vi "Run1TonNew.vi"() -> ()   [LabVIEW 2014]
doc: "Use this template to build a producer/consumer design pattern with events to produce queue items. Use this design pattern instead of the User Interface Event Handler pattern for user interfaces when you want to execute code asynchronously in response to an event without slowing the user interface responsiveness."
uses:
  <vilib>/addons/h5labview2/base/hid_t.ctl
  DatasetNames.ctl
  Program Files (x86)/CAEN/Comm/labview/CAENComm.lvlib
panel:
  out "Time Data (E-4 s)":T1
  in  "Monitoring Delay (ms)":u16=100 caption="Monitoring Delay (ms) (TDC, QDC, Dig, Time)"
  out "Duty Factor":dbl(graph)
  in  "?":T2(tab)
  out "TDC Histograms":u16[][](graph)
  out "QDC Histograms":u16[][](graph)
  out "Digitizer 1":dbl[][](graph)
  out "Scaler Rates":T3(graph)
  in  "Scaler Delay (s)":sgl=10.0
  out "Time Histogram":u16[][](graph)
  in  "Max Hist Time (s)":sgl=0.25 format="%#_13g"
  in  "Time # Bins":i32=1000
  out "Temp Chart":dynamicdata(graph)
  out "Total Samples":sgl caption="Number of Samples Being Averaged"
  out "Mean":sgl
  in  "Temp Delay (s)":sgl=1.0
  in  "Max Samples":u32=600
  out "# elements in queue":i32
  out "Acquiring?":bool
  out "Scaler Data":u32[](array[numeric])
  out "Acquisition\nErrors":errorcluster
  in  "Clear Acquisition Errors":bool
  in  "QDC threshold":u16=1
  in  "Start Acquisition":bool
  out "# Events Written":i32
  in  "# Events to\nRecord":i32
  out "Analysis\nErrors":errorcluster
  in  "Calibrate Verniers":bool
  in  "Stop Acquisition":bool
  in  "Configure Output":bool
  in  "Calibrate Pedestals":bool
  in  "stop":bool
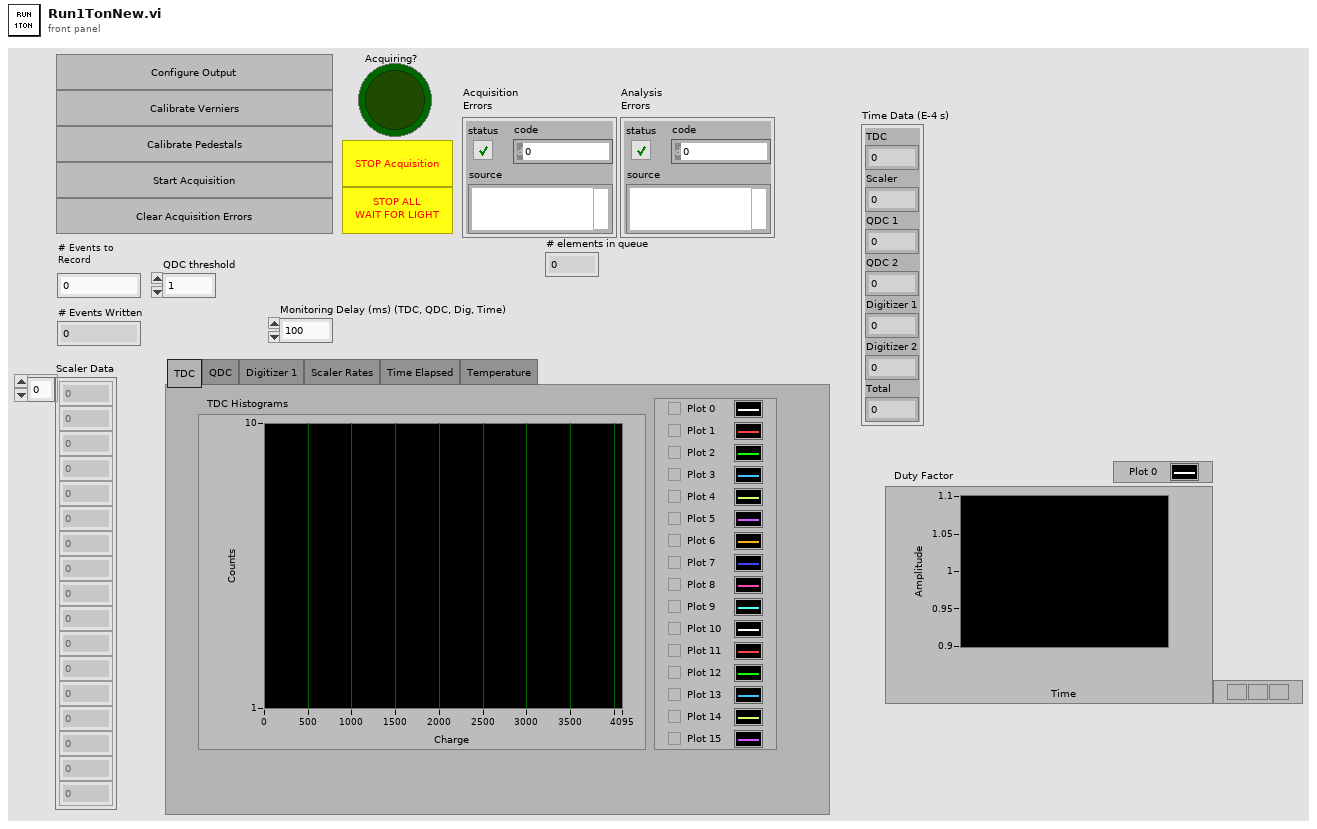
[diagram p1: front panel]
types:
  T1 = cluster{"TDC":u16, "Scaler":u16, "QDC 1":u16, "QDC 2":u16, "Digitizer 1":u16, "Digitizer 2":u16, "Total":u16}
  T2 = enum32{"TDC", "QDC", "Digitizer 1", "Scaler Rates", "Time Elapsed", "Temperature"}
  T3 = cluster{"[0]":dbl, "[1]":dbl, "[2]":dbl, "[3]":dbl}
  T4 = typedef "hid_t.ctl" = i32
  T5 = cluster{"State":enum16{"Startup", "Initialise", "Event OK", "Discard Event", "Exit", "Close"}, "Data":variant}
  T6 = typedef "DatasetNames.ctl" = enum16{"TDC", "Scaler", "QDC_1", "QDC_2", "Digitizer_1", "Digitizer_2", "Event_Time", "Event_Temp"}
  T7 = cluster{"TDC Data":u32[], "Scaler Data":u32[], "QDC 1 Data":u32[], "QDC 2 Data":u32[], "Digitizer 1 TRIG_REC":u32, "Digitizer 1 Waveforms":u32[], "Digitizer 2 TRIG_REC":u32, "Digitizer 2 Waveforms":u32[], "Event Start UNIX Time":dbl}
  T8 = enum16{"Startup", "Initialise", "Event OK", "Discard Event", "Exit", "Close"}
  T9 = cluster{"[0]":dbl, "[1]":dbl, "[2]":dbl, "[3]":dbl}[]
  T10 = cluster{"Channel":u8, "QDC Data":u16, "LowRange?":bool}[]
  T11 = cluster{"Data out[0]":u16, "Data out[1]":u16, "Data out[2]":u16, "Data out[3]":u16, "Data out[4]":u16, "Data out[5]":u16, "Data out[6]":u16}
  T12 = enum16{"Configure", "Initialise", "Run", "Close"}
  T13 = cluster{"TDC":u32, "Scaler":u32, "QDC 1":u32, "QDC 2":u32, "Digitizer 1":u32, "Digitizer 2":u32}
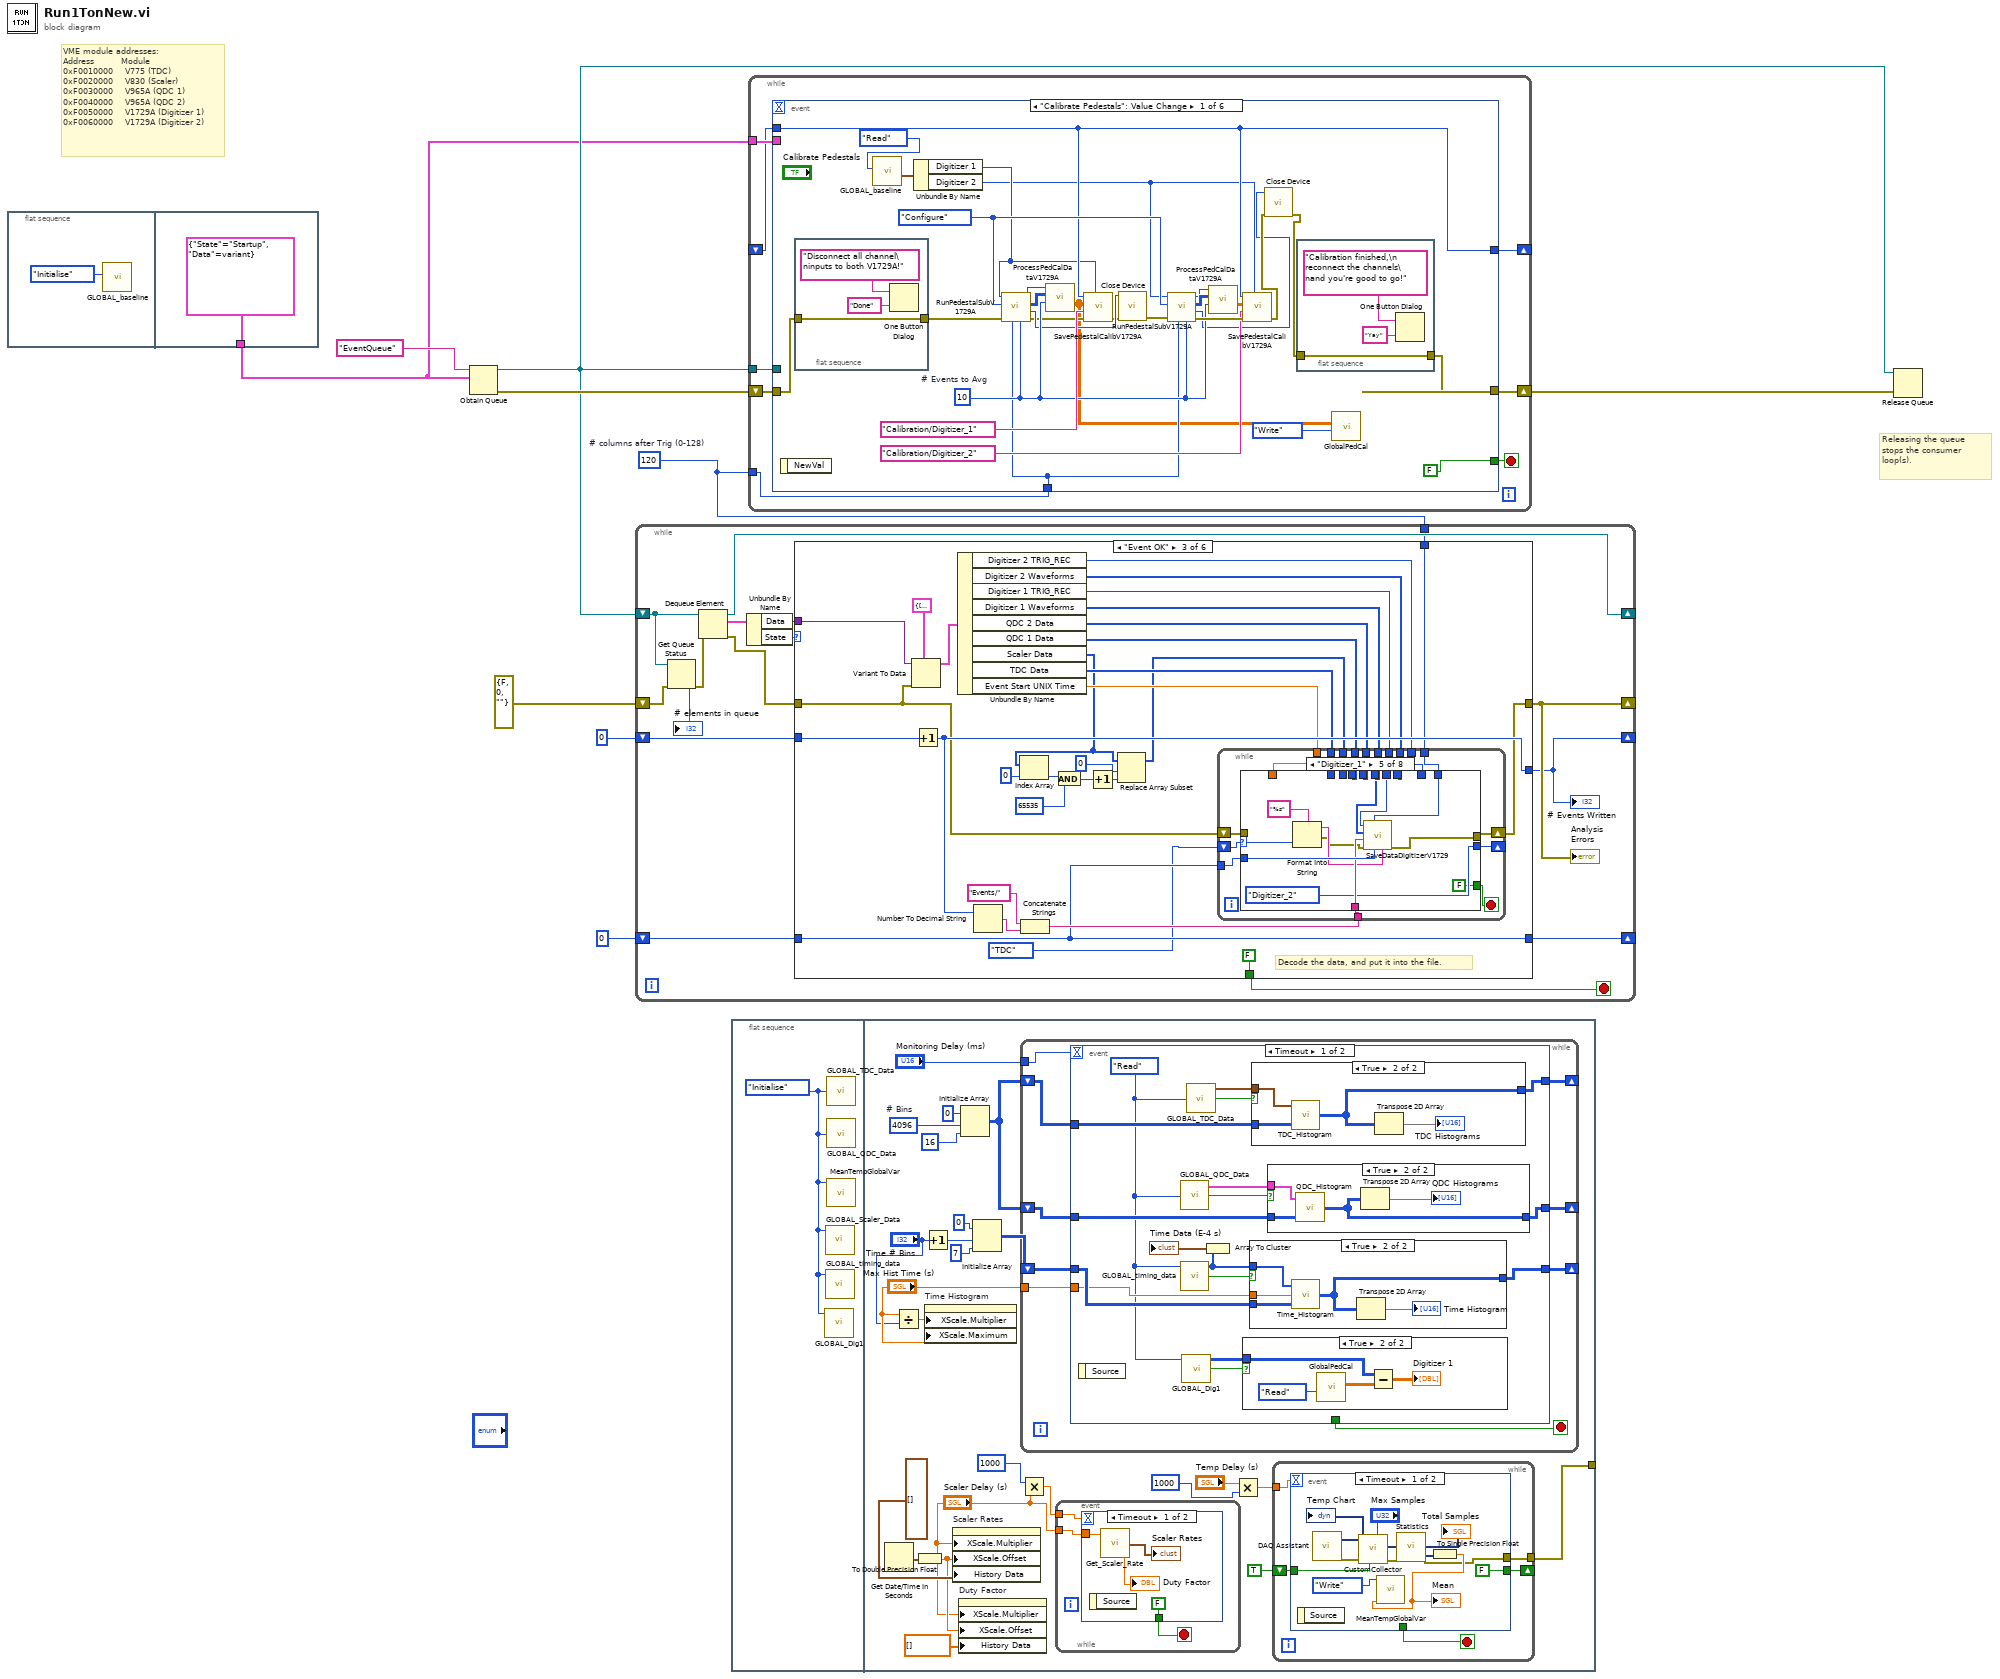
[diagram p0: block diagram]
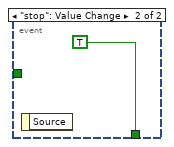
[diagram p2: hidden frame]
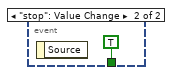
[diagram p3: hidden frame]
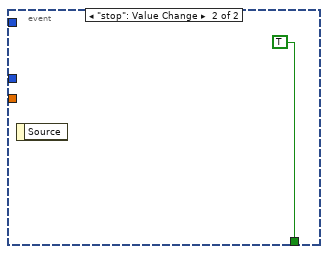
[diagram p8: hidden frame]
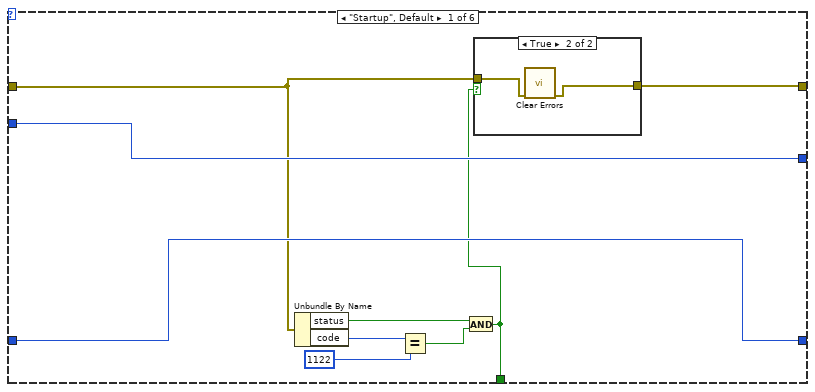
[diagram p9: hidden frame]
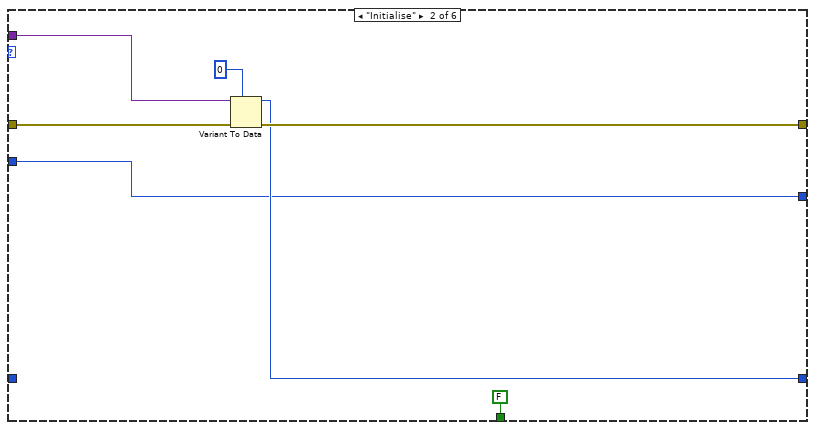
[diagram p11: hidden frame]
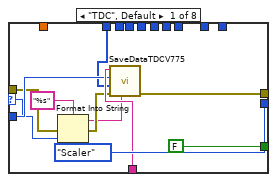
[diagram p12: hidden frame]
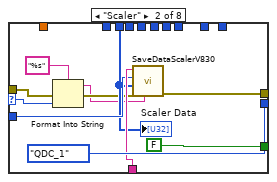
[diagram p13: hidden frame]
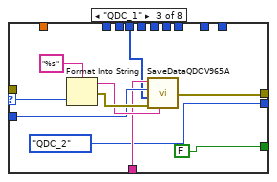
[diagram p14: hidden frame]
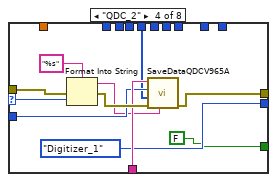
[diagram p15: hidden frame]
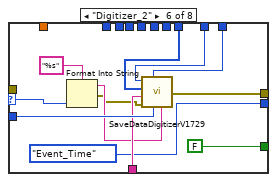
[diagram p16: hidden frame]
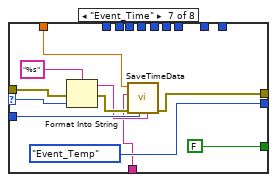
[diagram p17: hidden frame]
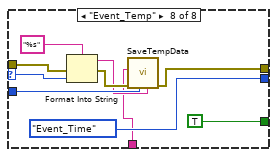
[diagram p18: hidden frame]
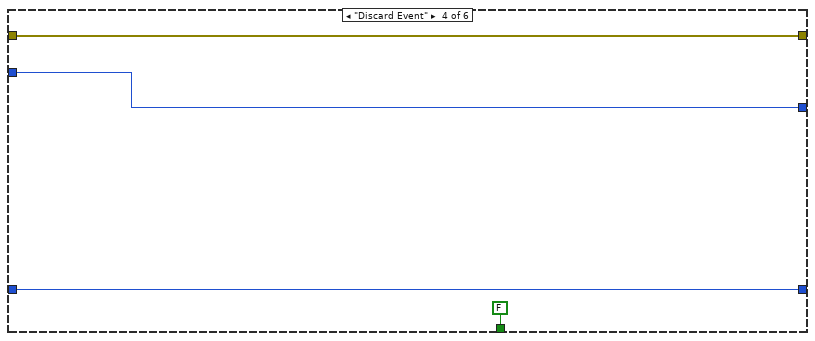
[diagram p19: hidden frame]
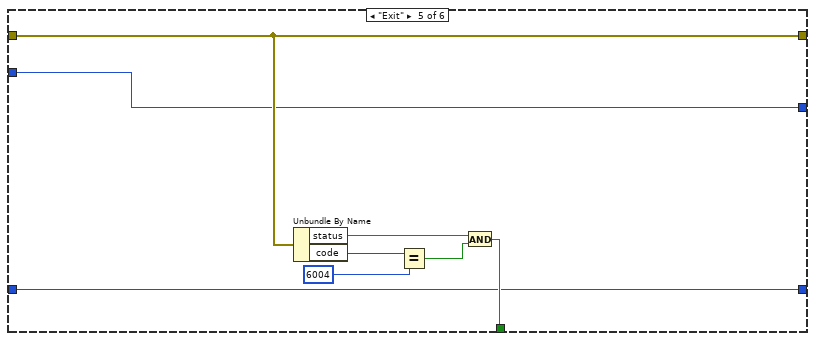
[diagram p20: hidden frame]
diagram:
  w1 = u16 120  # # columns after Trig (0-128)
  # "VME module addresses:\nAddress         Module\n0xF0010000    V775 (TDC)\n0xF0020000    V830 (Scaler)\n0xF0030000    V965A (QDC 1)\n0xF0040000    V965A (QDC 2)\n0xF0050000    V1729A (Digitizer 1)\n0xF0060000    V1729A (Digitizer 2)"
  # "Releasing the queue stops the consumer loop(s)."
  n1 = flat-sequence {
    tunnel: [T5 {"State"=enum."Startup", "Data"=variant}] -> w2
    frame #0 {
      n2 = call "GLOBAL_baseline.vi"("State"=enum16{"Initialise", "Write", "Read"}."Initialise") -> ()  [unwired: 10 in, 1 out]
    }
    frame #1 {
    }
  }
  n3 = Obtain Queue(name (unnamed)="EventQueue", element data type=w2) -> (queue out=w4:refnum<queue>, error out=w9:errorcluster)  [unwired: 3 in, 1 out]
  n4 = while {
    shift-right: [w17] -> _
    shift-left: errorcluster {"status"=FALSE, "code"=0, "source"=""} ("error out") -> [w15]
    shift-right: [w23] -> _
    shift-left: w4 -> [w13]
    shift-right: [w21] -> _
    shift-left: T4 0 ("File Handle") -> [w20]
    tunnel: w1 -> [w19]
    shift-right: [w16] -> _
    shift-left: 0 -> [w18]
    stop <- w22 stop-if-true
    n5 = Get Queue Status(queue=w13, error in (no error)=w15) -> (error out=w14:errorcluster, # elements in queue=→"# elements in queue":i32)  [unwired: 1 in, 6 out]
    n6 = Dequeue Element(queue=w13, error in (no error)=w14) -> (queue out=w23:refnum<queue>, element=w27:T5, error out=w24:errorcluster)  [unwired: 1 in, 1 out]
    n7 = Unbundle By Name(w27) -> ("Data"=w25:variant, "State"=w26:T8)
    n8 = case shown="\"Event OK\"" w26 {
      tunnel: w25 -> [_ w44 w75 _ _ _]
      tunnel: w24 -> [w30 w43 w62 w185 w188 w197]
      tunnel: [w28 w42 w60 w185 w188 w197] -> w17
      tunnel: [w29 FALSE FALSE FALSE w189 FALSE] -> w22
      tunnel: [w32 w41 w65 w183 w187 w195] -> w21
      tunnel: w20 -> [w32 _ w65 w183 w187 w195]
      tunnel: w19 -> [_ _ w67 _ _ _]
      tunnel: w18 -> [w31 w40 w74 w182 w186 w194]
      tunnel: [w31 w40 w73 w182 w186 w194] -> w16
      frame "Startup", Default {
        n9 = Unbundle By Name(w30) -> ("status"=w36:bool, "code"=w34:i32)
        n10 = Equal?(x=w34, y=1122) -> (x = y?=w35:bool)
        n11 = And(x=w36, y=w35) -> (x .and. y?=w29:bool)
        n12 = case shown="True" w29 {
          tunnel: w30 -> [w37 w39]
          tunnel: [w37 w38] -> w28
          frame False {
          }
          frame True {
            n13 = call <vilib>:"Clear Errors.vi"("error in (no error)"=w39) -> ("error out"=w38:errorcluster)  [unwired: 5 in, 1 out]
          }
        }
      }
      frame "Initialise" {
        n14 = Variant To Data(error in=w43, type=T4 0 ("File Handle"), Variant=w44) -> (data=w41:T4, error out=w42:errorcluster)
      }
      frame "Event OK" {
        # "Decode the data, and put it into the file."
        n15 = Variant To Data(error in=w62, type=T7 {"TDC Data"=[], "Scaler Data"=[], "QDC 1 Data"=[], "QDC 2 Data"=[], "Digitizer 1 TRIG_REC"=0, "Digitizer 1 Waveforms"=[], "Digitizer 2 TRIG_REC"=0, "Digitizer 2 Waveforms"=[], "Event Start UNIX Time"=0.0}, Variant=w75) -> (data=w69:T7)  [unwired: 1 out]
        n16 = Increment(x=w74) -> (x+1=w73:i32)
        n17 = Unbundle By Name(w69) -> ("Digitizer 2 TRIG_REC"=w68:u32, "Digitizer 2 Waveforms"=w55:u32[], "Digitizer 1 TRIG_REC"=w57:u32, "Digitizer 1 Waveforms"=w58:u32[], "QDC 2 Data"=w64:u32[], "QDC 1 Data"=w63:u32[], "Scaler Data"=w51:u32[], "TDC Data"=w61:u32[], "Event Start UNIX Time"=w56:dbl)
        n18 = Number To Decimal String(number=w73) -> (decimal integer string=w71:string)  [unwired: 1 in]
        n19 = Index Array(array=w51, index=0) -> (element=w53:u32)
        n20 = Concatenate Strings("Events/", w71) -> (w66:string)
        n21 = And(x=w53, y=u32 65535) -> (x .and. y?=w50:u32)
        n22 = Increment(x=w50) -> (x+1=w47:u32)
        n23 = Replace Array Subset(array=w51, new element=w47, index=0) -> (w48:u32[])
        n24 = while {
          tunnel: w68 -> [w93]
          tunnel: w55 -> [w92]
          tunnel: w67 -> [w91]
          tunnel: w66 -> [w90]
          tunnel: w65 -> [w89]
          tunnel: w57 -> [w88]
          tunnel: w58 -> [w87]
          tunnel: w64 -> [w85]
          tunnel: w63 -> [w84]
          shift-right: [w81] -> w60
          shift-left: w62 -> [w86]
          tunnel: w48 -> [w83]
          tunnel: w61 -> [w82]
          shift-right: [w80] -> _
          shift-left: DatasetNames."TDC" -> [w79]
          tunnel: w56 -> [w77]
          stop <- w78 stop-if-true
          n25 = case shown="\"Digitizer_1\"" w79 {
            selector: w79 -> [w94 w108 w122 w135 w144 w153 w170 w180]
            tunnel: [w102 w113 w119 w128 w148 w160 w164 w174] -> w81
            tunnel: w93 -> [_ _ _ _ _ w159 _ _]
            tunnel: w92 -> [_ _ _ _ _ w158 _ _]
            tunnel: w89 -> [w100 w111 w121 w131 w147 w157 w165 w175]
            tunnel: w91 -> [_ _ _ _ w146 w156 _ _]
            tunnel: w90 -> [w101 w112 w120 w132 w145 w155 w162 w172]
            tunnel: w88 -> [_ _ _ _ w140 _ _ _]
            tunnel: w87 -> [_ _ _ _ w139 _ _ _]
            tunnel: w86 -> [w97 w107 _ w134 _ _ w167 w177]
            tunnel: w85 -> [_ _ _ w130 _ _ _ _]
            tunnel: w84 -> [_ _ w118 _ _ _ _ _]
            tunnel: [DatasetNames."Scaler" DatasetNames."QDC_1" DatasetNames."QDC_2" DatasetNames."Digitizer_1" DatasetNames."Digitizer_2" DatasetNames."Event_Time" DatasetNames."Event_Temp" DatasetNames."Event_Time"] -> w80
            tunnel: [FALSE FALSE FALSE FALSE FALSE FALSE FALSE TRUE] -> w78
            tunnel: w83 -> [_ w110 _ _ _ _ _ _]
            tunnel: w82 -> [w99 _ _ _ _ _ _ _]
            tunnel: w77 -> [_ _ _ _ _ _ w161 _]
            frame "TDC", Default {
              n26 = Format Into String(format string="%s", error in=w97, w94) -> (resulting string=w95:string, error out=w96:errorcluster)  [unwired: 1 in]
              n27 = call "SaveDataTDCV775.vi"("Module"=w95, "error in (no error)"=w96, "Buff"=w99, "File Handle"=w100, "String"=w101) -> ("error out"=w102:errorcluster)  [unwired: 5 in, 1 out]
            }
            frame "Scaler" {
              n28 = Format Into String(format string="%s", error in=w107, w108) -> (resulting string=w105:string, error out=w106:errorcluster)  [unwired: 1 in]
              n29 = call "SaveDataScalerV830.vi"("Module"=w105, "error in (no error)"=w106, "Buff"=w110, "File Handle"=w111, "Group Name"=w112) -> ("error out"=w113:errorcluster)  [unwired: 6 in]
              "Scaler Data" <- w110
            }
            frame "QDC_1" {
              n30 = Format Into String(format string="%s", w122) -> (resulting string=w123:string, error out=w124:errorcluster)  [unwired: 2 in]
              n31 = call "SaveDataQDCV965A.vi"("Module"=w123, "error in (no error)"=w124, "Buff"=w118, "File Handle"=w121, "String"=w120) -> ("error out"=w119:errorcluster)  [unwired: 5 in, 1 out]
            }
            frame "QDC_2" {
              n32 = Format Into String(format string="%s", error in=w134, w135) -> (resulting string=w129:string, error out=w133:errorcluster)  [unwired: 1 in]
              n33 = call "SaveDataQDCV965A.vi"("Module"=w129, "error in (no error)"=w133, "Buff"=w130, "File Handle"=w131, "String"=w132) -> ("error out"=w128:errorcluster)  [unwired: 5 in, 1 out]
            }
            frame "Digitizer_1" {
              n34 = Format Into String(format string="%s", w144) -> (resulting string=w142:string, error out=w141:errorcluster)  [unwired: 2 in]
              n35 = call "SaveDataDigitizerV1729.vi"("Module"=w142, "File Handle"=w147, "# Samples after Trig"=w146, "error in (no error)"=w141, "String"=w145, "Digitizer Waveforms"=w139, "Digitizer TRIG_REC"=w140) -> ("error out"=w148:errorcluster)  [unwired: 2 in, 2 out]
            }
            frame "Digitizer_2" {
              n36 = Format Into String(format string="%s", w153) -> (resulting string=w152:string, error out=w151:errorcluster)  [unwired: 2 in]
              n37 = call "SaveDataDigitizerV1729.vi"("Module"=w152, "File Handle"=w157, "# Samples after Trig"=w156, "error in (no error)"=w151, "String"=w155, "Digitizer Waveforms"=w158, "Digitizer TRIG_REC"=w159) -> ("error out"=w160:errorcluster)  [unwired: 2 in, 2 out]
            }
            frame "Event_Time" {
              n38 = Format Into String(format string="%s", error in=w167, w170) -> (resulting string=w163:string, error out=w166:errorcluster)  [unwired: 1 in]
              n39 = call "SaveTimeData.vi"("Module"=w163, "File Handle"=w165, "error in (no error)"=w166, "String"=w162, "Event Start UNIX Time"=w161) -> ("error out"=w164:errorcluster)  [unwired: 5 in, 1 out]
            }
            frame "Event_Temp" {
              n40 = Format Into String(format string="%s", error in=w177, w180) -> (resulting string=w173:string, error out=w176:errorcluster)  [unwired: 1 in]
              n41 = call "SaveTempData.vi"("Module"=w173, "File Handle"=w175, "error in (no error)"=w176, "String"=w172) -> ("error out"=w174:errorcluster)  [unwired: 6 in, 1 out]
            }
          }
        }
      }
      frame "Discard Event" {
      }
      frame "Exit" {
        n42 = Unbundle By Name(w188) -> ("status"=w193:bool, "code"=w191:i32)
        n43 = Equal?(x=w191, y=6004) -> (x = y?=w192:bool)
        n44 = And(x=w193, y=w192) -> (x .and. y?=w189:bool)
      }
      frame "Close" {
      }
    }
    "Analysis\nErrors" <- w17
    "# Events Written" <- w16
  }
  n45 = flat-sequence {
    tunnel: [w199] -> _
    frame #0 {
      w198 = enum16{"Initialise", "Write", "Read"}."Initialise" ("State")
      n46 = call "GLOBAL_Dig1.vi"("State"=w198) -> ()  [unwired: 3 in, 2 out]
      n47 = call "GLOBAL_Scaler_Data.vi"("State"=w198) -> ()  [unwired: 4 in, 1 out]
      n48 = call "GLOBAL_timing_data.vi"("State"=w198) -> ()  [unwired: 3 in, 2 out]
      n49 = call "GLOBAL_TDC_Data.vi"("State"=w198) -> ()  [unwired: 3 in, 2 out]
      n50 = call "GLOBAL_QDC_Data.vi"("State"=w198) -> ()  [unwired: 3 in, 2 out]
      n51 = call "MeanTempGlobalVar.vi"("State"=w198) -> ()  [unwired: 10 in, 1 out]
    }
    frame #1 {
      w221 = u16 4096  # # Bins
      n52 = Get Date/Time In Seconds() -> (seconds since 1Jan1904=w218:timestamp)
      n53 = Divide(x="Max Hist Time (s)", y="Time # Bins") -> (x/y=w213:sgl)
      n54 = To Double Precision Float(number=w218) -> (double precision float=w209:dbl)
      n55 = Increment(x="Time # Bins") -> (x+1=w211:i32)
      n56 = property on="Time Histogram" class="WFGraph (strict)"("XScale.Multiplier"=w213, "XScale.Maximum"="Max Hist Time (s)") -> ()  [unwired: 2 in, 2 out]
      n57 = property on="Scaler Rates" class="WFChart (strict)"("XScale.Multiplier"="Scaler Delay (s)", "XScale.Offset"=w209, "History Data"=T9 []) -> ()  [unwired: 2 in, 2 out]
      n58 = property on="Duty Factor" class="WFChart (strict)"("XScale.Multiplier"="Scaler Delay (s)", "XScale.Offset"=w209, "History Data"=dbl[] []) -> ()  [unwired: 2 in, 2 out]
      n59 = Initialize Array(u16 0 ("element"), w221, 16 ("dimension size")) -> (w219:u16[][])
      n60 = Initialize Array(u16 0 ("element"), w211, 7 ("dimension size")) -> (w214:u16[][])
      n61 = Multiply(x=u32 1000 ("y"), y="Scaler Delay (s)") -> (x*y=w204:sgl)
      n62 = while {
        shift-right: [w251] -> _
        shift-left: w219 -> [w256]
        shift-right: [w253] -> _
        shift-left: w219 -> [w255]
        shift-right: [w252] -> _
        shift-left: w214 -> [w254]
        tunnel: "Max Hist Time (s)" -> [w257]
        tunnel: "Monitoring Delay (ms)" -> [w249]
        stop <- w250 stop-if-true
        n63 = event shown="[0] Timeout" {
          selector: _ -> [_ _]
          dyn-events: _ -> [_ _]
          timeout: w249 -> [_ _]
          tunnel: w257 -> [w266 _]
          tunnel: w256 -> [w269 _]
          tunnel: w255 -> [w268 _]
          tunnel: w254 -> [w267 _]
          tunnel: [w265 _] -> w253
          tunnel: [w264 _] -> w252
          tunnel: [w263 _] -> w251
          tunnel: [_ TRUE] -> w250
          event Timeout {
            w259 = enum16{"Initialise", "Write", "Read"}."Read" ("State")
            n64 = event-data() -> ()  [unwired: 1 in, 1 out]
            n65 = call "GLOBAL_QDC_Data.vi"("State"=w259) -> ("Valid Read?"=w272:bool, "Data Out"=w271:T10)  [unwired: 3 in]
            n66 = call "GLOBAL_timing_data.vi"("State"=w259) -> ("Valid Read?"=w270:bool, "Data out"=w262:u16[])  [unwired: 3 in]
            n67 = call "GLOBAL_Dig1.vi"("State"=w259) -> ("Valid Read?"=w260:bool, "Data Out"=w258:u16[][])  [unwired: 3 in]
            n68 = call "GLOBAL_TDC_Data.vi"("State"=w259) -> ("Valid Read?"=w274:bool, "Data Out"=w273:cluster{"Channel":u8, "TDC Data":u16}[])  [unwired: 3 in]
            n69 = Array To Cluster(array=w262) -> (cluster=→"Time Data (E-4 s)":T11)
            n70 = case shown="True" w260 {
              tunnel: w258 -> [_ w276]
              frame False {
              }
              frame True {
                n71 = call "GlobalPedCal.vi"("State"=enum16{"Initialise", "Write", "Read"}."Read") -> ("Data Out"=w277:dbl[][])  [unwired: 10 in]
                n72 = Subtract(x=w276, y=w277) -> (x-y=→"Digitizer 1":dbl[][])
              }
            }
            n73 = case shown="True" w270 {
              tunnel: w262 -> [_ w294]
              tunnel: [w289 w292] -> w264
              tunnel: w267 -> [w289 w291]
              tunnel: w266 -> [_ w290]
              frame False {
              }
              frame True {
                n74 = call "Time_Histogram.vi"("Hist array in"=w291, "Max (s)"=w290, "Data in"=w294) -> ("Hist array out"=w292:u16[][])  [unwired: 2 in]
                n75 = Transpose 2D Array(2D array=w292) -> (transposed array=→"Time Histogram":u16[][])
              }
            }
            n76 = case shown="True" w274 {
              tunnel: w273 -> [_ w288]
              tunnel: [w284 w286] -> w263
              tunnel: w269 -> [w284 w285]
              frame False {
              }
              frame True {
                n77 = call "TDC_Histogram.vi"("Hist array in"=w285, "Data In"=w288) -> ("Hist array out"=w286:u16[][])  [unwired: 3 in]
                n78 = Transpose 2D Array(2D array=w286) -> (transposed array=→"TDC Histograms":u16[][])
              }
            }
            n79 = case shown="True" w272 {
              tunnel: w271 -> [_ w283]
              tunnel: [w279 w281] -> w265
              tunnel: w268 -> [w279 w280]
              frame False {
              }
              frame True {
                n80 = call "QDC_Histogram.vi"("Hist array in"=w280, "Data In"=w283) -> ("Hist array out"=w281:u16[][])  [unwired: 3 in]
                n81 = Transpose 2D Array(2D array=w281) -> (transposed array=→"QDC Histograms":u16[][])
              }
            }
          }
          event "stop": Value Change {
            n82 = event-data() -> ()  [unwired: 1 in, 1 out]
          }
        }
      }
      n83 = while {
        tunnel: "Scaler Delay (s)" -> [w242]
        tunnel: w204 -> [w241]
        stop <- w243 stop-if-true
        n84 = event shown="[0] Timeout" {
          selector: _ -> [_ _]
          dyn-events: _ -> [_ _]
          timeout: w241 -> [_ _]
          tunnel: w242 -> [w247 _]
          tunnel: [FALSE TRUE] -> w243
          event Timeout {
            n85 = event-data() -> ()  [unwired: 1 in, 1 out]
            n86 = call "Get_Scaler_Rate.vi"("Delay Time (s)"=w247) -> ("Duty Factor"=→"Duty Factor":dbl, "Cluster out"=→"Scaler Rates":T3)  [unwired: 3 in]
          }
          event "stop": Value Change {
            n87 = event-data() -> ()  [unwired: 1 in, 1 out]
          }
        }
      }
      n88 = Multiply(x="Temp Delay (s)", y=u16 1000) -> (x*y=w206:sgl)
      n89 = while {
        shift-right: [w227] -> _
        shift-left: TRUE -> [w225]
        tunnel: w206 -> [w224]
        tunnel: [w223] -> w199
        stop <- w226 stop-if-true
        n90 = event shown="[0] Timeout" {
          selector: _ -> [_ _]
          dyn-events: _ -> [_ _]
          timeout: w224 -> [_ _]
          tunnel: [FALSE _] -> w227
          tunnel: w225 -> [w228 _]
          tunnel: [_ TRUE] -> w226
          tunnel: [w229 _] -> w223
          event Timeout {
            n91 = event-data() -> ()  [unwired: 1 in, 1 out]
            n92 = call "DAQ Assistant"() -> ("data"=w232:dynamicdata, "error out"=w238:errorcluster)  [unwired: 17 in, 1 out]
            "Temp Chart" <- w232
            n93 = call "CustomCollector.vi"("Reset"=w228, "error in (no error)"=w238, "Size"="Max Samples", "Signals"=w232) -> ("error out"=w237:errorcluster, "Collected Signals"=w239:dynamicdata)  [unwired: 6 in]
            n94 = call "Statistics"("Signals"=w239, "error in (no error)"=w237) -> ("Total Samples"=→"Total Samples":dynamicdata, "Arithmetic Mean"=w235:dynamicdata, "error out"=w229:errorcluster)  [unwired: 23 in]
            n95 = To Single Precision Float(number=w235) -> (single precision float=w234:sgl)
            "Mean" <- w234
            n96 = call "MeanTempGlobalVar.vi"("Temp In"=w234, "State"=enum16{"Initialise", "Write", "Read"}."Write") -> ()  [unwired: 9 in, 1 out]
          }
          event "stop": Value Change {
            n97 = event-data() -> ()  [unwired: 1 in, 1 out]
          }
        }
      }
    }
  }
  n98 = while {
    shift-right: [w301] -> w6
    shift-left: w9 -> [w302]
    tunnel: w4 -> [w303]
    tunnel: w2 -> [w299]
    tunnel: w1 -> [w298]
    shift-right: [w297] -> _
    shift-left: _ -> [w296]
    stop <- w300 stop-if-true
    n99 = event shown="[0] \"Calibrate Pedestals\": Value Change" {
      selector: _ -> [_ _ _ _ _ _]
      dyn-events: _ -> [_ _ _ _ _ _]
      timeout: _ -> [_ _ _ _ _ _]
      tunnel: w303 -> [_ _ _ w346 w359 _]
      tunnel: w302 -> [w307 w341 _ w347 w361 w489]
      tunnel: [w327 w341 _ w350 _ w488] -> w301
      tunnel: [FALSE ("stop") "stop" FALSE ("stop") FALSE ("stop") FALSE ("stop") _] -> w300
      tunnel: w299 -> [_ _ _ w351 w360 _]
      tunnel: w298 -> [w320 _ _ _ w356 _]
      tunnel: [w326 w340 w342 w344 w355 _] -> w297
      tunnel: w296 -> [w326 w340 w342 _ w355 _]
      event "Calibrate Pedestals": Value Change {
        w330 = T12."Configure"
        w321 = 10  # # Events to Avg
        n100 = event-data() -> ()  [unwired: 1 in, 1 out]
        n101 = flat-sequence {
          tunnel: w307 -> [w338]
          tunnel: [w338] -> w317
          frame #0 {
            n102 = One Button Dialog(message="Disconnect all channel\ninputs to both V1729A!", button name ("OK")="Done") -> ()  [unwired: 1 out]
          }
        }
        n103 = call "GLOBAL_baseline.vi"("State"=enum16{"Initialise", "Write", "Read"}."Read") -> ("Addresses Out"=w324:T13)  [unwired: 10 in]
        n104 = Unbundle By Name(w324) -> ("Digitizer 1"=w316:u32, "Digitizer 2"=w313:u32)
        n105 = call "RunPedestalSubV1729A.vi"("# Events to Avg"=w321, "# Samples after Trig"=w320, "error in (no error)"=w317, "Init State"=w330, "VME Base Address in"=w316) -> ("error out"=w310:errorcluster, "handle out"=w315:i32, "Data Out"=w331:u32[][], "Offset"=w309:i16)  [unwired: 3 in]
        n106 = call "ProcessPedCalDataV1729A.vi"("# Events to Avg"=w321, "Data In"=w331, "Offset"=w309) -> ("Channel Data"=w304:dbl[][])  [unwired: 8 in]
        n107 = call "SavePedestalCalibV1729A.vi"("Address"=w316, "error in (no error)"=w310, "Group Name"="Calibration/Digitizer_1", "Data In"=w304, "File Handle"=w326) -> ("error out"=w312:errorcluster)  [unwired: 6 in]
        n108 = call "Close Device.vi"("error in (no error)"=w312, "handle"=w315) -> ("error out"=w311:errorcluster)  [unwired: 9 in]
        n109 = call "RunPedestalSubV1729A.vi"("# Events to Avg"=w321, "# Samples after Trig"=w320, "error in (no error)"=w311, "Init State"=w330, "VME Base Address in"=w313) -> ("error out"=w328:errorcluster, "handle out"=w314:i32, "Data Out"=w329:u32[][], "Offset"=w308:i16)  [unwired: 3 in]
        n110 = call "ProcessPedCalDataV1729A.vi"("# Events to Avg"=w321, "Data In"=w329, "Offset"=w308) -> ("Channel Data"=w305:dbl[][])  [unwired: 8 in]
        n111 = call "SavePedestalCalibV1729A.vi"("Address"=w313, "error in (no error)"=w328, "Group Name"="Calibration/Digitizer_2", "Data In"=w305, "File Handle"=w326) -> ("error out"=w319:errorcluster)  [unwired: 6 in]
        n112 = call "Close Device.vi"("error in (no error)"=w319, "handle"=w314) -> ("error out"=w318:errorcluster)  [unwired: 9 in]
        n113 = flat-sequence {
          tunnel: w318 -> [w333]
          tunnel: [w333] -> w327
          frame #0 {
            n114 = One Button Dialog(message="Calibration finished,\n reconnect the channels\nand you're good to go!", button name ("OK")="Yay") -> ()  [unwired: 1 out]
          }
        }
        n115 = call "GlobalPedCal.vi"("State"=enum16{"Initialise", "Write", "Read"}."Write", "Data In"=w304) -> ()  [unwired: 9 in, 1 out]
      }
      event "stop": Value Change {
        n116 = event-data() -> ()  [unwired: 1 in, 1 out]
      }
      event "Calibrate Verniers": Value Change {
        # "This needs to be implemented if we want better timing resolution on the digitizers (apparently ~70 ps)\n- The user will need to feed in a sawtooth waveform.\n- This calibration will determine MINVER and MAXVER for each digitizer (see V1729A manual)\n- The MINVER and MAXVER correction can be applied offline (or online if we can spare the delay)."
        n117 = event-data() -> ()  [unwired: 1 in, 1 out]
      }
      event "Configure Output": Value Change {
        w352 = T8."Initialise"  # State
        n118 = event-data() -> ()  [unwired: 1 in, 1 out]
        n119 = call "CreateHDF5.vi"() -> ("error out"=w349:errorcluster, "File Handle"=w344:T4)  [unwired: 10 in]
        n120 = To Variant(anything=w344) -> (Variant=w353:variant)
        n121 = Bundle By Name(cluster=w351, "State"=w352, "Data"=w353) -> (w345:T5)
        n122 = Enqueue Element(queue=w346, element=w345, error in (no error)=w347) -> (error out=w348:errorcluster)  [unwired: 1 in, 2 out]
        n123 = Merge Errors(w349, w348) -> (w350:errorcluster)
      }
      event "Start Acquisition": Value Change {
        n124 = event-data() -> ()  [unwired: 1 in, 1 out]
        n125 = while {
          shift-right: [w372] -> _
          shift-left: T12."Configure" -> [w377]
          shift-right: [w375] -> _
          shift-left: w361 -> [w376]
          shift-right: [w374] -> _
          shift-left: _ -> [w373]
          tunnel: w360 -> [w371]
          tunnel: w359 -> [w370]
          tunnel: "# Events to\nRecord" -> [w368]
          shift-right: [w366] -> _
          shift-left: 0 -> [w369]
          tunnel: w356 -> [w365]
          stop <- w367 stop-if-true
          n126 = case shown="\"Run\"" w377 {
            tunnel: w376 -> [w418 w434 w466 w478]
            tunnel: [w403 w435 w460 w484] -> w375
            tunnel: [w402 w425 w440 w476] -> w374
            tunnel: w373 -> [_ w433 w440 w476]
            tunnel: [T12."Initialise" T12."Run" w457 T12."Close"] -> w372
            tunnel: w371 -> [_ _ w463 w480]
            tunnel: w370 -> [_ _ w462 w483]
            tunnel: w369 -> [w416 w436 w456 w485]
            tunnel: w368 -> [_ _ w455 _]
            tunnel: [_ _ _ TRUE] -> w367
            tunnel: [w416 w436 w453 w485] -> w366
            tunnel: w365 -> [w405 _ _ _]
            tunnel: [_ _ TRUE _] -> w364
            frame "Configure", Default {
              w394 = u16 32 ("High range threshold")
              w395 = TRUE ("Count only accepted trigs?\n(else all trigs)")
              w409 = u16 1 ("# Evts to Acquire")
              w404 = FALSE ("Software Trig?")
              n127 = call "GLOBAL_baseline.vi"("State"=enum16{"Initialise", "Write", "Read"}."Read") -> ("Addresses Out"=w389:T13)  [unwired: 10 in]
              n128 = call "OpenInterface.vi"("error in (no error)"=w418) -> ("error out"=w383:errorcluster, "handle"=w382:i32)  [unwired: 8 in, 1 out]
              n129 = Unbundle By Name(w389) -> ("Digitizer 2"=w384:u32, "Digitizer 1"=w385:u32, "QDC 2"=w386:u32, "QDC 1"=w387:u32, "Scaler"=w381:u32, "TDC"=w388:u32)
              n130 = call "ConfigureScaler.vi"("error in (no error)"=w383, "handle"=w382, "VME Base Address"=w381) -> ("error out"=w380:errorcluster, "handle out"=w378:i32)  [unwired: 6 in, 1 out]
              n131 = call "ConfigTDC.vi"("# Evts to Acquire"=w409, "Interrupt Level"=u16 1, "error in (no error)"=w380, "FSR setting"=u16 255, "handle"=w382, "VME Base Address"=w388) -> ("error out"=w413:errorcluster, "handle out"=w412:i32)  [unwired: 4 in]
              n132 = call "SetRangeTDC.vi"("Low Range threshold"=u16 1, "error in (no error)"=w413, "handle"=w412, "VME module Base Address"=w388) -> ("error out"=w379:errorcluster)  [unwired: 5 in, 2 out]
              n133 = call "ConfigureQDC.vi"("VME module Base Address"=w387, "IRQ Lvl"=u16 1, "handle"=w378, "error in (no error)"=w379, "# of events before transfer (max 32)"=w409) -> ("error out"=w401:errorcluster, "handle out"=w400:i32)  [unwired: 5 in]
              n134 = call "RangeAndSetupQDC.vi"("Count only accepted trigs?\n(else all trigs)"=w395, "VME module Base Address"=w387, "error in (no error)"=w401, "High range threshold"=w394, "handle in"=w400, "Low Range threshold"="QDC threshold") -> ("error out"=w399:errorcluster, "handle out"=w398:i32)  [unwired: 4 in]
              n135 = call "ConfigureQDC.vi"("VME module Base Address"=w386, "IRQ Lvl"=u16 2, "handle"=w398, "error in (no error)"=w399, "# of events before transfer (max 32)"=w409) -> ("error out"=w397:errorcluster, "handle out"=w392:i32)  [unwired: 5 in]
              n136 = call "RangeAndSetupQDC.vi"("Count only accepted trigs?\n(else all trigs)"=w395, "VME module Base Address"=w386, "error in (no error)"=w397, "High range threshold"=w394, "handle in"=w392, "Low Range threshold"="QDC threshold") -> ("error out"=w396:errorcluster, "handle out"=w391:i32)  [unwired: 4 in]
              n137 = call "ConfigureDigitizer_PedCal.vi"("Software Trig?"=w404, "error in (no error)"=w396, "# Samples after Trig"=w405, "handle"=w391, "VME Base Address"=w385) -> ("error out"=w407:errorcluster, "handle out"=w406:i32)  [unwired: 4 in, 1 out]
              n138 = call "ConfigureDigitizer_PedCal.vi"("Software Trig?"=w404, "error in (no error)"=w407, "# Samples after Trig"=w405, "handle"=w406, "VME Base Address"=w384) -> ("error out"=w403:errorcluster, "handle out"=w402:i32)  [unwired: 4 in, 1 out]
            }
            frame "Initialise" {
              n139 = call "GLOBAL_baseline.vi"("State"=enum16{"Initialise", "Write", "Read"}."Read") -> ("Addresses Out"=w423:T13)  [unwired: 10 in]
              n140 = Unbundle By Name(w423) -> ("QDC 2"=w419:u32, "QDC 1"=w420:u32, "Scaler"=w421:u32, "TDC"=w422:u32)
              n141 = call "ClearEventsTDC.vi"("error in (no error)"=w434, "handle"=w433, "VME module Base Address"=w422) -> ("error out"=w432:errorcluster, "handle out"=w431:i32)  [unwired: 6 in, 1 out]
              n142 = call "ClearEventsV830.vi"("error in (no error)"=w432, "handle in"=w431, "VME Base Address"=w421) -> ("error out"=w430:errorcluster, "handle out"=w429:i32)  [unwired: 7 in]
              n143 = call "ClearEventsQDC.vi"("error in (no error)"=w430, "handle"=w429, "VME module Base Address"=w420) -> ("error out"=w428:errorcluster, "handle out"=w427:i32)  [unwired: 6 in, 1 out]
              n144 = call "ClearEventsQDC.vi"("error in (no error)"=w428, "handle"=w427, "VME module Base Address"=w419) -> ("error out"=w426:errorcluster, "handle out"=w425:i32)  [unwired: 6 in, 1 out]
              n145 = call "IRQ Enable.vi"("error in (no error)"=w426, "handle"=w425) -> ("error out"=w435:errorcluster)  [unwired: 9 in]
            }
            frame "Run" {
              # "Acquire"
              n146 = call <vilib>:"Clear Errors.vi"("error in (no error)"=w466, "specific error code to clear (0: all)"=-7) -> ("error out"=w445:errorcluster)  [unwired: 4 in, 1 out]
              n147 = call "GLOBAL_baseline.vi"("State"=enum16{"Initialise", "Write", "Read"}."Read") -> ("Addresses Out"=w451:T13)  [unwired: 10 in]
              n148 = Unbundle By Name(w451) -> ("Digitizer 2"=w447:u32, "Digitizer 1"=w450:u32)
              n149 = call "AcquireEventDigitizerV1729A.vi"("error in (no error)"=w445, "handle in"=w440, "VME Base Address"=w450) -> ("error out"=w449:errorcluster, "handle out"=w448:i32)  [unwired: 7 in]
              n150 = Increment(x=w456) -> (x+1=w453:i32)
              n151 = call "AcquireEventDigitizerV1729A.vi"("error in (no error)"=w449, "handle in"=w448, "VME Base Address"=w447) -> ("error out"=w446:errorcluster)  [unwired: 7 in, 1 out]
              "Acquisition\nErrors" <- w446
              n152 = Greater Or Equal?(x=w453, y=w455) -> (x >= y?=w454:bool)
              n153 = while {
                tunnel: w446 -> [w473]
                tunnel: [w472] -> w438
                tunnel: w440 -> [w471]
                shift-right: [w470] -> _
                shift-left: u8 0 ("Mask") -> [w468]
                stop <- w467 stop-if-true
                n154 = Equal?(x=w468, y=u8 7) -> (x = y?=w467:bool)
                n155 = call "VMEIRQ Check.vi"("error in (no error)"=w473, "VMEhandle"=w471) -> ("error out"=w472:errorcluster, "Mask"=w470:u8)  [unwired: 8 in]
              }
              n156 = Or(x=w454, y="Stop Acquisition") -> (x .or. y?=w458:bool)
              n157 = call "GetAllData.vi"("error in (no error)"=w438, "handle in"=w440) -> ("error out"=w439:errorcluster, "Data cluster"=w443:T7)  [unwired: 7 in, 1 out]
              n158 = case shown="False" w458 {
                tunnel: [T12."Run" T12."Close"] -> w457
                frame False {
                }
                frame True {
                }
              }
              n159 = To Variant(anything=w443) -> (Variant=w465:variant)
              n160 = Bundle By Name(cluster=w463, "State"=T8."Event OK", "Data"=w465) -> (w461:T5)
              n161 = Enqueue Element(queue=w462, element=w461, error in (no error)=w439) -> (error out=w460:errorcluster)  [unwired: 1 in, 2 out]
            }
            frame "Close" {
              n162 = call "Close Device.vi"("error in (no error)"=w478, "handle"=w476) -> ("error out"=w477:errorcluster)  [unwired: 9 in]
              n163 = Bundle By Name(cluster=w480, "State"=T8."Close", "Data"=variant) -> (w479:T5)
              n164 = Enqueue Element(queue=w483, element=w479, error in (no error)=w477) -> (error out=w484:errorcluster)  [unwired: 1 in, 2 out]
            }
          }
          "Acquiring?" <- w364
        }
      }
      event "Clear Acquisition Errors": Value Change {
        n165 = event-data() -> ()  [unwired: 1 in, 2 out]
        n166 = call <vilib>:"Clear Errors.vi"("error in (no error)"=w489) -> ("error out"=w488:errorcluster)  [unwired: 5 in, 1 out]
      }
    }
  }
  n167 = Release Queue(queue=w4, error in (no error)=w6) -> ()  [unwired: 1 in, 3 out]
